vi "set insecure mode for tls config.vi"(8 "error in":errorcluster, 11 "config in":u64) -> (0 "error out":errorcluster)   [LabVIEW 2016, in "lv tls dll.lvlib"]
uses:
  lv tls dll.lvlib
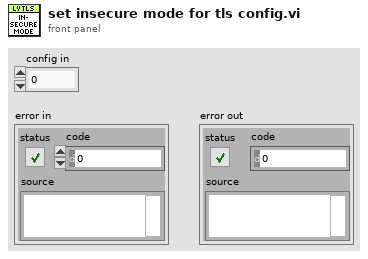
[diagram p1: front panel]
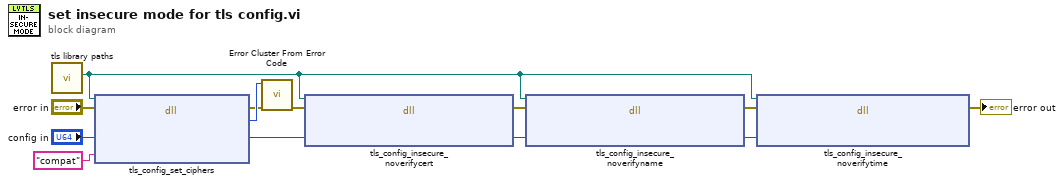
[diagram p0: block diagram]
diagram:
  n1 = call "tls library paths.vi"() -> ("libtls"=w1:path)  [unwired: 8 in, 3 out]
  n2 = dll-call lib="C:/Users/IEUser/Desktop/tlssimple/libtls-15.dll" fn="tls_config_set_ciphers"(path in=w1, error in="error in", "config"="config in", "ciphers"="compat") -> (error out=w6:errorcluster, "err"=w9:i32, "config"=w11:u64)  [unwired: 2 in, 1 out]
  n3 = call <vilib>:"Error Cluster From Error Code.vi"("error in (no error)"=w6, "error code (0)"=w9) -> ("error out"=w8:errorcluster)  [unwired: 7 in]
  n4 = dll-call lib="C:/Users/IEUser/Desktop/tlssimple/libtls-15.dll" fn="tls_config_insecure_noverifycert"(path in=w1, error in=w8, "config"=w11) -> (error out=w7:errorcluster, "config"=w10:u64)  [unwired: 2 in, 1 out]
  n5 = dll-call lib="C:/Users/IEUser/Desktop/tlssimple/libtls-15.dll" fn="tls_config_insecure_noverifyname"(path in=w1, error in=w7, "config"=w10) -> (error out=w4:errorcluster, "config"=w3:u64)  [unwired: 2 in, 1 out]
  n6 = dll-call lib="C:/Users/IEUser/Desktop/tlssimple/libtls-15.dll" fn="tls_config_insecure_noverifytime"(path in=w1, error in=w4, "config"=w3) -> (error out=→"error out":errorcluster)  [unwired: 3 in, 1 out]
